vi "Scanner_main_15_2D_2channels.vi"() -> ()   [LabVIEW 2016]
uses:
  <vilib>/DAQmx/write.llb/DAQmx Write (Digital Bool 1Line 1Point).vi
  <vilib>/DAQmx/read.llb/DAQmx Read (Analog 1D DBL 1Chan NSamp).vi
  <vilib>/DAQmx/write.llb/DAQmx Write (Analog 1D Wfm NChan NSamp).vi
  <vilib>/DAQmx/read.llb/DAQmx Read (Counter 1D DBL 1Chan NSamp).vi
  <vilib>/DAQmx/create/channels.llb/DAQmx Create Channel (AO-Voltage-Basic).vi
  <vilib>/DAQmx/configure/timing.llb/DAQmx Timing (Sample Clock).vi
  <vilib>/DAQmx/configure/trigger.llb/DAQmx Start Trigger (Digital Edge).vi
  <vilib>/DAQmx/create/channels.llb/DAQmx Create Channel (AI-Voltage-Basic).vi
  <vilib>/DAQmx/create/channels.llb/DAQmx Create Channel (CI-Count Edges).vi
  Global 1.vi
  <vilib>/DAQmx/miscellaneous.llb/DAQmx Fill In Error Info.vi
  <vilib>/DAQmx/create/channels.llb/DAQmx Create Channel (DO-Digital Output).vi
  <resource>/objmgr/daqmx.rc
panel:
  out "Refl":dbl[][](graph)
  out "Step (um)":dbl
  out "saved":bool
  in  "folder":path=path "C:/Users/Sergey/Scan"
  in  "filename":string="1"
  out "Scan_pix":i32
  out "Frame":dbl
  out "length of scan":i32
  in  "OK Button":bool
  in  "delta_p":i32=-24
  out "Line":i32
  in  "offset Y":dbl
  in  "offset X":dbl
  in  "stop":bool
  in  "Save":bool
  in  "Multi/Single":bool
  in  "Range":dbl=250.0
  in  "Pixels":i32=128
  in  "Dwell":dbl=5e-05 format="%#_6p"
  out "Fluorescence":i16[][](graph)
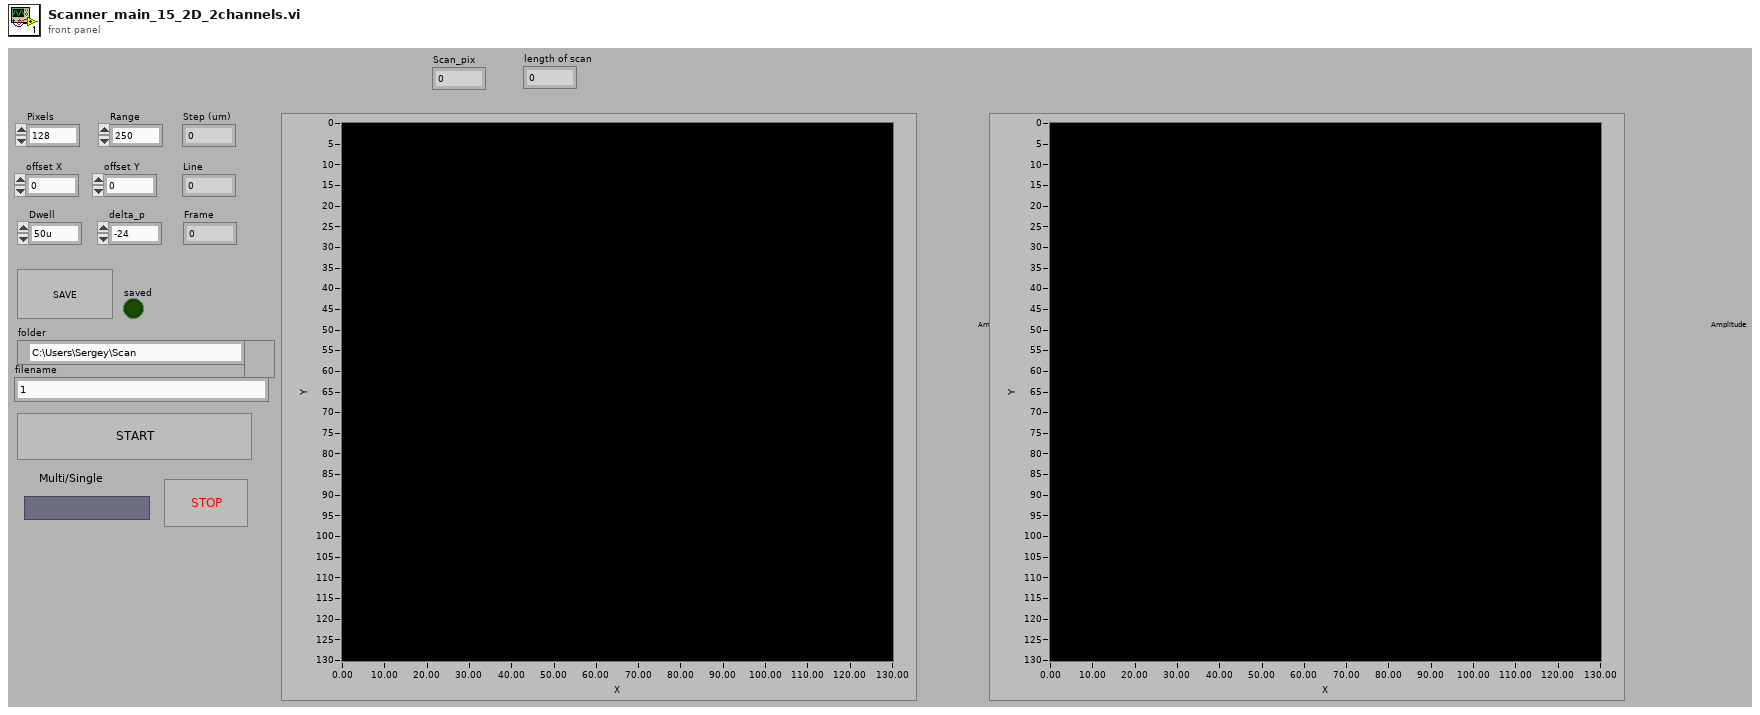
[diagram p1: front panel]
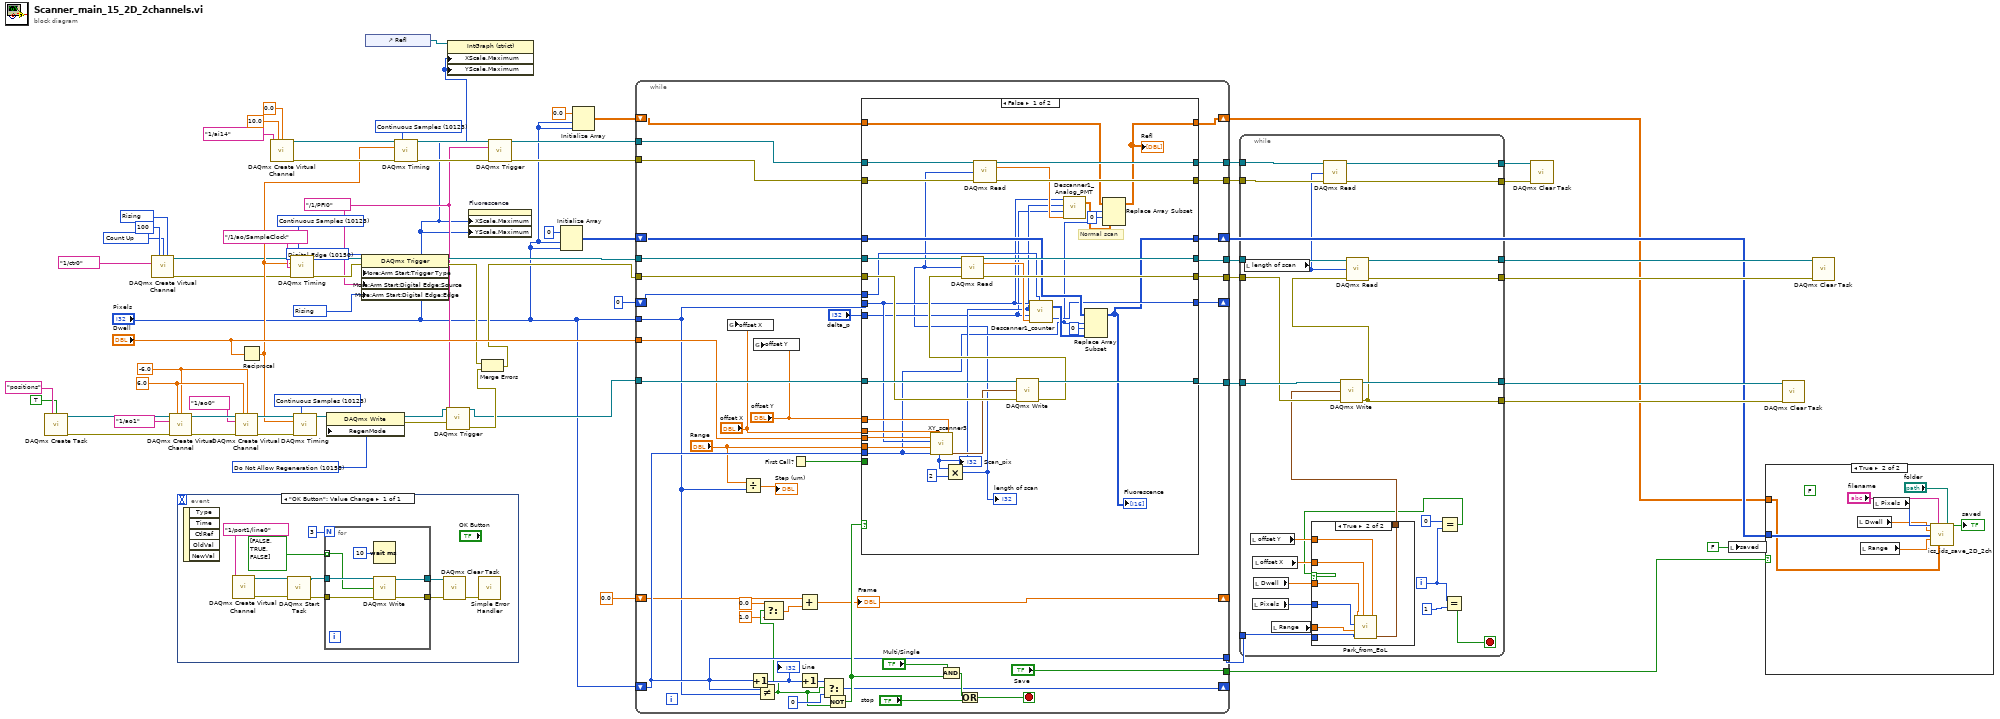
[diagram p0: block diagram]
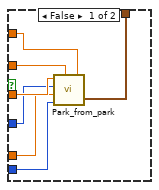
[diagram p2: hidden frame]
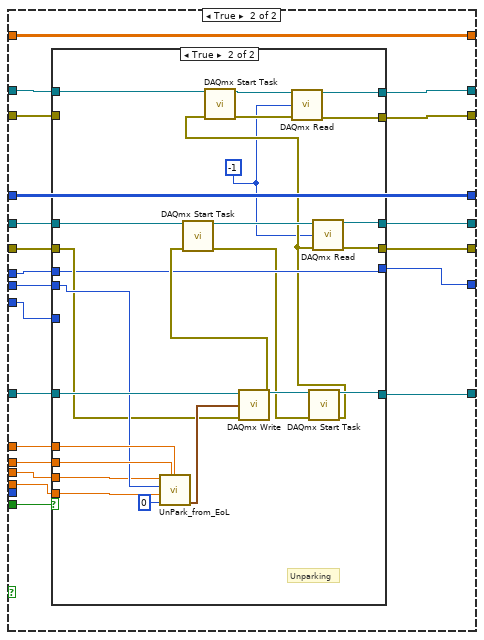
[diagram p4: hidden frame]
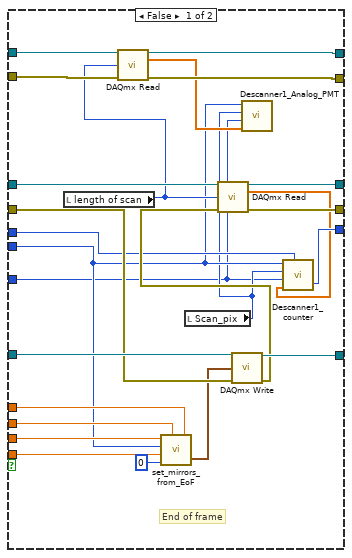
[diagram p5: hidden frame]
diagram:
  w4 = 10280 items=["Rising"=10280, "Falling"=10171] ("edge")
  w5 = 10128 items=["Count Up"=10128, "Count Down"=10124, "Externally Controlled"=10326] ("count direction")
  w25 = 10123 items=["Finite Samples"=10178, "Continuous Samples"=10123] ("sample mode")
  w45 = 10280 items=["Rising"=10280, "Falling"=10171] ("ArmStart.DigEdge.Edge")
  w17 = tag "/1/PFI0" ("ArmStart.DigEdge.Src")
  w46 = 10150 items=["Digital Edge"=10150, "None"=10230] ("ArmStart.TrigType")
  w59 = 10158 items=["Allow Regeneration"=10097, "Do Not Allow Regeneration"=10158] ("RegenMode")
  w63 = 6.0 ("maximum value")
  w62 = -6.0 ("minimum value")
  w69 = 10123 items=["Finite Samples"=10178, "Continuous Samples"=10123] ("sample mode")
  w71 = 10123 items=["Finite Samples"=10178, "Continuous Samples"=10123] ("sample mode")
  n1 = call <vilib>:"DAQmx Create Task.vi"("new task name"="positions", "auto cleanup"=TRUE) -> ("task out"=w55:refnum<k21>, "error out"=w52:errorcluster)  [unwired: 12 in]
  n2 = call-poly <vilib>:"DAQmx Create Virtual Channel.vi"("initial count"=u32 100, "count direction"=w5, "edge"=w4, "counter"=tag "1/ctr0") -> ("task out"=w3:refnum<k21>, "error out"=w6:errorcluster)  [unwired: 10 in]
  n3 = call-poly <vilib>:"DAQmx Create Virtual Channel.vi"("task in"=w55, "maximum value"=w63, "minimum value"=w62, "physical channels"=tag "1/ao1", "error in"=w52) -> ("task out"=w68:refnum<k21>, "error out"=w66:errorcluster)  [unwired: 9 in]
  n4 = event shown="[0] \"OK Button\": Value Change" {
    selector: _ -> [_]
    dyn-events: _ -> [_]
    timeout: _ -> [_]
    event "OK Button": Value Change {
      n5 = event-data() -> ()  [unwired: 6 out]
      n6 = call-poly <vilib>:"DAQmx Create Virtual Channel.vi"("lines"=tag "1/port1/line0" ("Software Trigger Line")) -> ("task out"=w80:refnum<k21>, "error out"=w79:errorcluster)  [unwired: 4 in, 9 out]
      n7 = call <vilib>:"DAQmx Start Task.vi"("task/channels in"=w80, "error in"=w79) -> ("task out"=w78:refnum<k21>, "error out"=w77:errorcluster)  [unwired: 12 out]
      n8 = for {
        N: 3 -> [_]
        tunnel: w78 -> [w86]
        tunnel: w77 -> [w85]
        tunnel: bool[] [FALSE, TRUE, FALSE] -> [w84] mode=indexing
        tunnel: [w83] -> w74
        tunnel: [w82] -> w73
        n9 = Wait (ms)(milliseconds to wait=u32 10) -> ()  [unwired: 1 out]
        n10 = call-poly <vilib>:"DAQmx Write.vi"("task/channels in"=w86, "data"=w84, "error in"=w85) -> ("task out"=w82:refnum<k21>, "error out"=w83:errorcluster)  [unwired: 1 in, 10 out]
      }
      n11 = call <vilib>:"DAQmx Clear Task.vi"("task in"=w73, "error in"=w74) -> ("error out"=w75:errorcluster)  [unwired: 13 out]
      n12 = call <vilib>:"Simple Error Handler.vi"("error in (no error)"=w75) -> ()  [unwired: 1 in, 8 out]
    }
  }
  n13 = call-poly <vilib>:"DAQmx Create Virtual Channel.vi"("task in"=w68, "maximum value"=w63, "minimum value"=w62, "physical channels"=tag "1/ao0" ("physical channels 2"), "error in"=w66) -> ("task out"=w67:refnum<k21>, "error out"=w65:errorcluster)  [unwired: 9 in]
  n14 = Reciprocal(x="Dwell") -> (1/x=w7:dbl)
  n15 = call-poly <vilib>:"DAQmx Create Virtual Channel.vi"("maximum value"=10.0, "minimum value"=0.0, "physical channels"=tag "1/ai14") -> ("task out"=w21:refnum<k21>, "error out"=w20:errorcluster)  [unwired: 11 in]
  n16 = call-poly <vilib>:"DAQmx Timing.vi"("task/channels in"=w3, "sample mode"=w71, "rate"=w7, "source"=tag "/1/ao/SampleClock", "error in"=w6) -> ("task out"=w48:refnum<k21>, "error out"=w47:errorcluster)  [unwired: 9 in]
  n17 = call-poly <vilib>:"DAQmx Timing.vi"("task/channels in"=w67, "sample mode"=w69, "rate"=w7, "error in"=w65) -> ("task out"=w61:refnum<k21>)  [unwired: 10 in, 1 out]
  n18 = property class="DAQmx Write"(reference=w61, "RegenMode"=w59) -> (reference out=w43:refnum<k21>, error out=w42:errorcluster)  [unwired: 1 in]
  n19 = property class="DAQmx Trigger"(reference=w48, error in=w47, "More:Arm Start:Trigger Type"=w46, "More:Arm Start:Digital Edge:Source"=w17, "More:Arm Start:Digital Edge:Edge"=w45) -> (reference out=w39:refnum<k21>, error out=w44:errorcluster)
  n20 = control-ref of="Refl"() -> (w2:refnum<vi>)
  n21 = call-poly <vilib>:"DAQmx Timing.vi"("task/channels in"=w21, "sample mode"=w25, "rate"=w7, "error in"=w20) -> ("task out"=w19:refnum<k21>, "error out"=w18:errorcluster)  [unwired: 10 in]
  n22 = call-poly <vilib>:"DAQmx Trigger.vi"("task/channels in"=w43, "source"=w17, "error in"=w42) -> ("task out"=w40:refnum<k21>, "error out"=w41:errorcluster)  [unwired: 11 in]
  n23 = property on="Property Node" class="IntGraph (strict)"(reference=w2, "XScale.Maximum"="Pixels", "YScale.Maximum"="Pixels") -> ()  [unwired: 1 in, 2 out]
  n24 = property on="Fluorescence" class="IntGraph (strict)"("XScale.Maximum"="Pixels", "YScale.Maximum"="Pixels") -> ()  [unwired: 2 in, 2 out]
  n25 = Merge Errors(w44, w41) -> (w38:errorcluster)
  n26 = call-poly <vilib>:"DAQmx Trigger.vi"("task/channels in"=w19, "source"=w17, "error in"=w18) -> ("task out"=w16:refnum<k21>, "error out"=w15:errorcluster)  [unwired: 11 in]
  n27 = Initialize Array(i16 0 ("element"), "Pixels", "Pixels") -> (w57:i16[][])
  n28 = Initialize Array(0.0 ("element"), "Pixels", "Pixels") -> (w13:dbl[][])
  n29 = while {
    tunnel: w40 -> [w117]
    tunnel: w39 -> [w113]
    tunnel: w38 -> [w112]
    tunnel: "Pixels" -> [w97]
    tunnel: "Dwell" -> [w111]
    shift-right: [w108] -> _
    shift-left: "Pixels" -> [w107]
    tunnel: [w120] -> w35
    shift-right: [w114] -> w27
    shift-left: w57 -> [w115]
    tunnel: ["Save"] -> w56
    tunnel: [w119] -> w36
    tunnel: [w118] -> w37
    tunnel: [w107] -> w30
    shift-right: [w101] -> _
    shift-left: 0.0 ("t") -> [w102]
    shift-right: [w99] -> _
    shift-left: 0 ("t") -> [w100]
    tunnel: w16 -> [w93]
    tunnel: w15 -> [w92]
    tunnel: [w91] -> w12
    tunnel: [w90] -> w11
    shift-right: [w89] -> w8
    shift-left: w13 -> [w88]
    stop <- w109 stop-if-true
    n30 = global write "Global 1.vi" "offset X"("offset X") -> ()
    n31 = Divide(x="Range", y=w97) -> (x/y=→"Step (um)":dbl)
    n32 = Increment(x=w107) -> (x+1=w124:i32)
    "Line" <- w124
    n33 = global write "Global 1.vi" "offset Y"("offset Y") -> ()
    n34 = Not Equal?(x=w107, y=w97) -> (x != y?=w105:bool)
    n35 = Select(t=0.0, s=w105, f=1.0) -> (s? t:f=w106:dbl)
    n36 = First Call?() -> (First Call?: T/F=w110:bool)
    n37 = Add(x=w102, y=w106) -> (x+y=w101:dbl)
    "Frame" <- w101
    n38 = Increment(x=w124) -> (x+1=w122:i32)
    n39 = Select(t=w122, s=w105, f=0) -> (s? t:f=w108:i32)
    n40 = Not(x=w105) -> (.not. x?=w121:bool)
    n41 = case shown="False" w121 {
      tunnel: [w159 w182] -> w119
      tunnel: w113 -> [w160 w183]
      tunnel: [w158 w179] -> w120
      tunnel: w112 -> [w149 w178]
      tunnel: [w161 w180] -> w118
      tunnel: w117 -> [w162 w181]
      tunnel: "delta_p" -> [w135 w168]
      tunnel: w97 -> [w137 w171]
      tunnel: w115 -> [w157 w177]
      tunnel: [w143 w177] -> w114
      tunnel: "offset Y" -> [w155 w176]
      tunnel: "offset X" -> [w154 w175]
      tunnel: w111 -> [w153 w174]
      tunnel: "Range" -> [w152 w173]
      tunnel: w107 -> [w134 _]
      tunnel: w110 -> [_ w172]
      tunnel: w100 -> [w146 w169]
      tunnel: [w145 w170] -> w99
      tunnel: w93 -> [w142 w167]
      tunnel: w92 -> [w141 w166]
      tunnel: [w140 w165] -> w91
      tunnel: [w139 w164] -> w90
      tunnel: [w131 w163] -> w89
      tunnel: w88 -> [w130 w163]
      frame False {
        # "Normal scan"
        n42 = call "XY_scanner3.vi"("offset Y"=w155, "offset X"=w154, "Line_start"=w134, "Range"=w152, "Pixels"=w137, "dwell"=w153) -> ("X and Y"=w147:waveform(dbl)[], "scanPix"=w136:i32)  [unwired: 2 out]
        "Scan_pix" <- w136
        n43 = Multiply(x=w136, y=2) -> (x*y=w129:i32)
        "length of scan" <- w129
        n44 = call-poly <vilib>:"DAQmx Read.vi"("task/channels in"=w142, "number of samples per channel"=w129, "error in"=w141) -> ("task out"=w140:refnum<k21>, "data"=w138:dbl[], "error out"=w139:errorcluster)  [unwired: 10 in]
        n45 = call-poly <vilib>:"DAQmx Write.vi"("task/channels in"=w162, "data"=w147, "error in"=w149) -> ("task out"=w161:refnum<k21>, "error out"=w150:errorcluster)  [unwired: 10 in, 1 out]
        n46 = call-poly <vilib>:"DAQmx Read.vi"("task/channels in"=w160, "number of samples per channel"=w129, "error in"=w150) -> ("task out"=w159:refnum<k21>, "data"=w144:dbl[], "error out"=w158:errorcluster)  [unwired: 10 in]
        n47 = call "Descanner1_counter.vi"("Pix"=w137, "scanPix"=w136, "delta_p"=w135, "Data"=w144, "last_count prev line"=w146) -> ("2Lines"=w148:i64[][], "last_count"=w145:i64)
        n48 = call "Descanner1_Analog_PMT.vi"("Pix"=w137, "scanPix"=w136, "delta_p"=w135, "Data"=w138) -> ("2Lines"=w132:dbl[][])  [unwired: 2 in]
        n49 = Replace Array Subset(array=w157, new element=w148, index (row)=w134, index (col)=0 ("disabled index (col)")) -> (w143:i16[][])
        "Fluorescence" <- w143
        n50 = Replace Array Subset(array=w130, new element=w132, index (row)=w134, index (col)=0 ("disabled index (col)")) -> (w131:dbl[][])
        "Refl" <- w131
      }
      frame True {
        n51 = case shown="True" w172 {
          tunnel: w183 -> [w208 w222]
          tunnel: [w207 w218] -> w182
          tunnel: w181 -> [w206 w233]
          tunnel: [w205 w224] -> w180
          tunnel: [w203 w217] -> w179
          tunnel: w171 -> [w186 w230]
          tunnel: w178 -> [w201 w223]
          tunnel: w176 -> [w198 w232]
          tunnel: w175 -> [w197 w231]
          tunnel: w174 -> [w200 w229]
          tunnel: w173 -> [w196 w228]
          tunnel: [w194 w220] -> w170
          tunnel: w169 -> [w195 w220]
          tunnel: w168 -> [w184 _]
          tunnel: w167 -> [w192 w214]
          tunnel: w166 -> [w191 _]
          tunnel: [w189 w210] -> w165
          tunnel: [w188 w209] -> w164
          frame False {
            # "End of frame"
            n52 = local read "length of scan"() -> (w190:i32)
            n53 = call-poly <vilib>:"DAQmx Read.vi"("task/channels in"=w192, "number of samples per channel"=w190, "error in"=w191) -> ("task out"=w189:refnum<k21>, "data"=w187:dbl[], "error out"=w188:errorcluster)  [unwired: 10 in]
            n54 = call "set_mirrors_from_EoF.vi"("offset Y"=w198, "offset X"=w197, "Line_start"=0, "Range"=w196, "Pixels"=w186, "dwell"=w200) -> ("X and Y"=w199:waveform(dbl)[])  [unwired: 1 out]
            n55 = local read "Scan_pix"() -> (w185:i32)
            n56 = call-poly <vilib>:"DAQmx Write.vi"("task/channels in"=w206, "data"=w199, "error in"=w201) -> ("task out"=w205:refnum<k21>, "error out"=w204:errorcluster)  [unwired: 10 in, 1 out]
            n57 = call-poly <vilib>:"DAQmx Read.vi"("task/channels in"=w208, "number of samples per channel"=w190, "error in"=w204) -> ("task out"=w207:refnum<k21>, "data"=w193:dbl[], "error out"=w203:errorcluster)  [unwired: 10 in]
            n58 = call "Descanner1_Analog_PMT.vi"("Pix"=w186, "scanPix"=w185, "delta_p"=w184, "Data"=w187) -> ()  [unwired: 2 in, 1 out]
            n59 = call "Descanner1_counter.vi"("Pix"=w186, "scanPix"=w185, "delta_p"=w184, "Data"=w193, "last_count prev line"=w195) -> ("last_count"=w194:i64)  [unwired: 1 out]
          }
          frame True {
            w211 = -1 ("number of samples per channel")
            # "Unparking"
            n60 = call "UnPark_from_EoL.vi"("offset Y"=w232, "offset X"=w231, "Line_start"=0, "Range"=w228, "Pixels"=w230, "dwell"=w229) -> ("X and Y"=w226:waveform(dbl)[])  [unwired: 2 out]
            n61 = call-poly <vilib>:"DAQmx Write.vi"("task/channels in"=w233, "data"=w226, "error in"=w223) -> ("task out"=w225:refnum<k21>, "error out"=w221:errorcluster)  [unwired: 10 in, 1 out]
            n62 = call <vilib>:"DAQmx Start Task.vi"("task/channels in"=w222, "error in"=w221) -> ("task out"=w219:refnum<k21>, "error out"=w216:errorcluster)  [unwired: 12 in]
            n63 = call <vilib>:"DAQmx Start Task.vi"("task/channels in"=w225, "error in"=w216) -> ("task out"=w224:refnum<k21>, "error out"=w215:errorcluster)  [unwired: 12 in]
            n64 = call <vilib>:"DAQmx Start Task.vi"("task/channels in"=w214, "error in"=w215) -> ("task out"=w213:refnum<k21>, "error out"=w212:errorcluster)  [unwired: 12 in]
            n65 = call-poly <vilib>:"DAQmx Read.vi"("task/channels in"=w213, "number of samples per channel"=w211, "error in"=w212) -> ("task out"=w210:refnum<k21>, "error out"=w209:errorcluster)  [unwired: 10 in, 1 out]
            n66 = call-poly <vilib>:"DAQmx Read.vi"("task/channels in"=w219, "number of samples per channel"=w211, "error in"=w215) -> ("task out"=w218:refnum<k21>, "error out"=w217:errorcluster)  [unwired: 10 in, 1 out]
          }
        }
      }
    }
    n67 = And(x="Multi/Single", y=w121) -> (x .and. y?=w125:bool)
    n68 = Or(x=w125, y="stop") -> (x .or. y?=w109:bool)
  }
  n69 = while {
    tunnel: w37 -> [w257]
    tunnel: w30 -> [w256]
    tunnel: w36 -> [w255]
    tunnel: w35 -> [w254]
    tunnel: [w253] -> w32
    tunnel: [w252] -> w34
    tunnel: [w245] -> w33
    tunnel: [w251] -> w31
    tunnel: w12 -> [w238]
    tunnel: w11 -> [w237]
    tunnel: [w235] -> w10
    tunnel: [w234] -> w9
    i -> [w241]
    stop <- w244 stop-if-true
    n70 = local read "length of scan"() -> (w236:i32)
    n71 = local read "offset Y"() -> (w248:dbl)
    n72 = local read "Pixels"() -> (w242:i32)
    n73 = local read "offset X"() -> (w247:dbl)
    n74 = local read "Dwell"() -> (w249:dbl)
    n75 = local read "Range"() -> (w250:dbl)
    n76 = call-poly <vilib>:"DAQmx Read.vi"("task/channels in"=w238, "number of samples per channel"=w236, "error in"=w237) -> ("task out"=w235:refnum<k21>, "error out"=w234:errorcluster)  [unwired: 10 in, 1 out]
    n77 = Equal?(x=0, y=w241) -> (x = y?=w239:bool)
    n78 = case shown="True" w239 {
      tunnel: w256 -> [w260 w265]
      tunnel: w250 -> [w261 w266]
      tunnel: w249 -> [w263 w268]
      tunnel: w248 -> [w258 w270]
      tunnel: w247 -> [w259 w269]
      tunnel: [w264 w271] -> w246
      tunnel: w242 -> [w262 w267]
      frame False {
        n79 = call "Park_from_park.vi"("offset Y"=w258, "offset X"=w259, "Line_start"=w260, "Range"=w261, "Pixels"=w262, "dwell"=w263) -> ("X and Y"=w264:waveform(dbl)[])  [unwired: 1 in]
      }
      frame True {
        n80 = call "Park_from_EoL.vi"("offset Y"=w270, "offset X"=w269, "Line_start"=w265, "Range"=w266, "Pixels"=w267, "dwell"=w268) -> ("X and Y"=w271:waveform(dbl)[])  [unwired: 1 in, 2 out]
      }
    }
    n81 = call-poly <vilib>:"DAQmx Write.vi"("task/channels in"=w257, "data"=w246, "error in"=w254) -> ("task out"=w253:refnum<k21>, "error out"=w251:errorcluster)  [unwired: 10 in, 1 out]
    n82 = call-poly <vilib>:"DAQmx Read.vi"("task/channels in"=w255, "number of samples per channel"=w236, "error in"=w251) -> ("task out"=w252:refnum<k21>, "error out"=w245:errorcluster)  [unwired: 10 in, 1 out]
    n83 = Equal?(x=w241, y=1) -> (x = y?=w244:bool)
  }
  n84 = call <vilib>:"DAQmx Clear Task.vi"("task in"=w10, "error in"=w9) -> ()  [unwired: 13 in, 1 out]
  n85 = local write "saved"(FALSE ("saved")) -> ()
  n86 = case shown="True" w56 {
    tunnel: w27 -> [_ w279]
    tunnel: w8 -> [_ w272]
    frame False {
    }
    frame True {
      (unwired) FALSE ("prepend array or string size? (T)")
      n87 = local read "Dwell"() -> (w277:dbl)
      n88 = local read "Range"() -> (w276:dbl)
      n89 = local read "Pixels"() -> (w278:i32)
      n90 = call "ics_ids_save_2D_2ch.vi"("pixels 2"=w278, "filename 2"="filename", "folder 2"="folder", "Dwell 2"=w277, "data"=w279, "Range 2"=w276, "data 2"=w272) -> ("saved"=→"saved":bool)  [unwired: 7 in, 1 out]
    }
  }
  n91 = call <vilib>:"DAQmx Clear Task.vi"("task in"=w32, "error in"=w31) -> ()  [unwired: 13 in, 1 out]
  n92 = call <vilib>:"DAQmx Clear Task.vi"("task in"=w34, "error in"=w33) -> ()  [unwired: 13 in, 1 out]
